vi "Post_Process_Profile_Remote.vi"(1 "Results Plotter Rows":string[][](array[string]), 2 "Raw Data files to PP":path[](array[path]), 3 "Current Results filenames":path[](array[path])) -> ()   [LabVIEW 2010]
uses:
  Globals/Constants_global.vi
panel:
  in  "User Specific":refnum<vi>
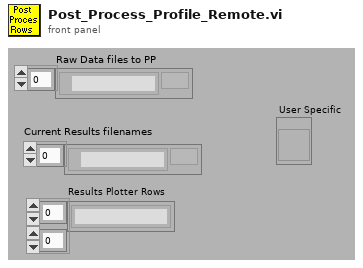
[diagram p1: front panel]
types:
  T1 = enum32{"Bad", "Idle", "Run top level", "Running"}
  T2 = enum16{"A single file", "Original Results Filenames with _PP", "Current Results Filenames"}
  T3 = enum16{"Left Button", "Center Button", "Right Button", "Window Close"}
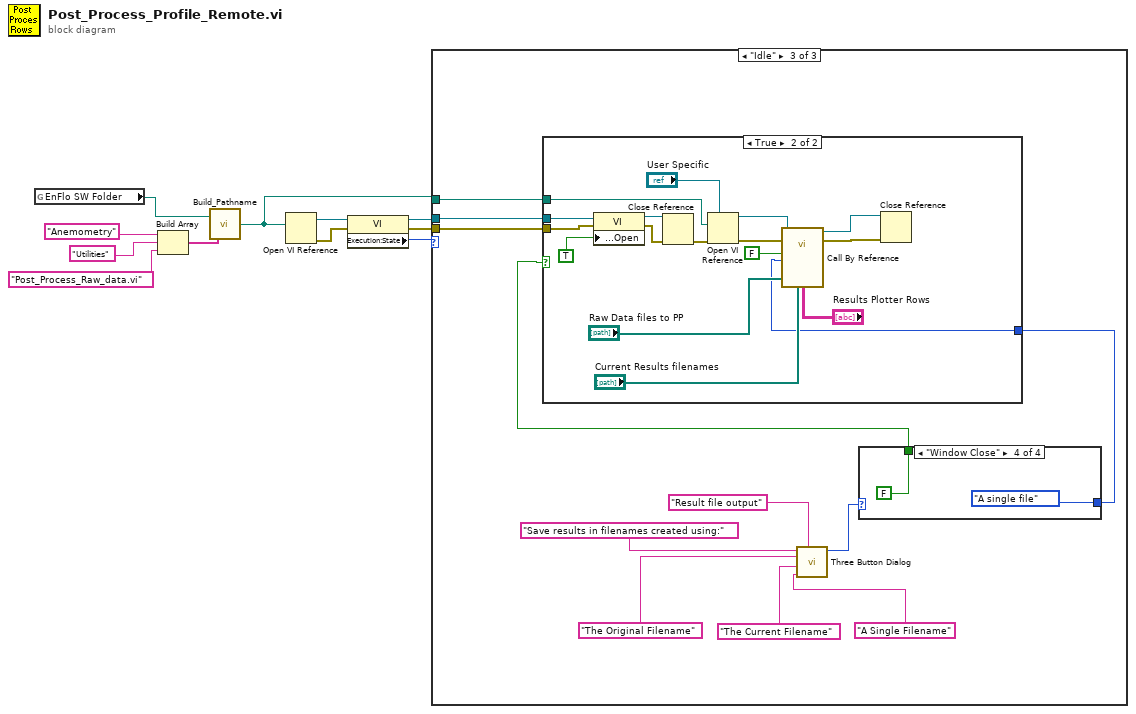
[diagram p0: block diagram]
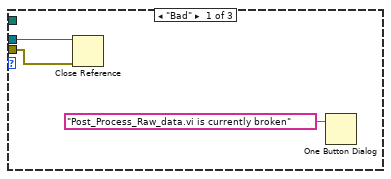
[diagram p2: hidden frame]
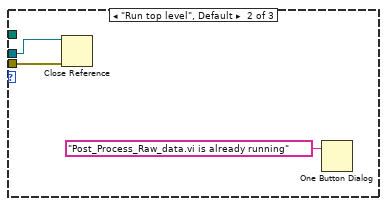
[diagram p3: hidden frame]
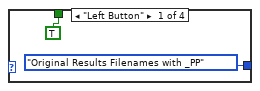
[diagram p5: hidden frame]
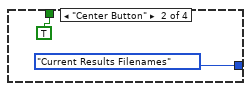
[diagram p6: hidden frame]
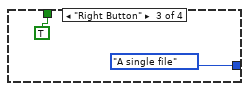
[diagram p7: hidden frame]
diagram:
  n1 = global read "Constants_global.vi" "EnFlo SW Folder"() -> (w11:path)
  n2 = Build Array("Anemometry", "Utilities", "Post_Process_Raw_data.vi") -> (w10:string[])
  n3 = call "Build_Pathname.vi"("Output Array"=w10, "Pathname"=w11) -> ("Appended path"=w2:path)
  n4 = Open VI Reference(vi path=w2) -> (vi reference=w6:refnum<vi>, error out=w7:errorcluster)  [unwired: 1 in, 4 out]
  n5 = property class="VI"(reference=w6, error in=w7) -> (reference out=w4:refnum<vi>, error out=w3:errorcluster, "Execution:State"=w5:T1)
  n6 = case shown="\"Idle\"" w5 {
    tunnel: w4 -> [w13 w16 w28]
    tunnel: w3 -> [w12 w15 w27]
    tunnel: w2 -> [_ _ w26]
    frame "Bad" {
      n7 = Close Reference(reference=w13, error in (no error)=w12) -> ()  [unwired: 1 out]
      n8 = One Button Dialog(message="Post_Process_Raw_data.vi is currently broken") -> ()  [unwired: 2 out]
    }
    frame "Run top level", Default {
      n9 = Close Reference(reference=w16, error in (no error)=w15) -> ()  [unwired: 1 out]
      n10 = One Button Dialog(message="Post_Process_Raw_data.vi is already running") -> ()  [unwired: 2 out]
    }
    frame "Idle" {
      n11 = call <vilib>:"Three Button Dialog.vi"("Window Title (\"\")"="Result file output" ("Window Title (\"\")"), "Right Button Text (\"Cancel\")"="A Single Filename" ("Left Button Text (\"Yes\")"), "Center Button Text (\"No\")"="The Current Filename" ("Left Button Text (\"Yes\")"), "Left Button Text (\"Yes\")"="The Original Filename" ("Left Button Text (\"Yes\")"), "message"="Save results in filenames created using:") -> ("Which Button?"=w20:T3)  [unwired: 6 out]
      n12 = case shown="\"Window Close\"" w20 {
        tunnel: [T2."Original Results Filenames with _PP" ("Save results to") T2."Current Results Filenames" ("Save results to") T2."A single file" ("Save results to") T2."A single file" ("Save results to")] -> w19
        tunnel: [TRUE TRUE TRUE FALSE] -> w18
        frame "Left Button" {
        }
        frame "Center Button" {
        }
        frame "Right Button" {
        }
        frame "Window Close" {
        }
      }
      n13 = case shown="True" w18 {
        tunnel: w28 -> [_ w45]
        tunnel: w27 -> [_ w44]
        tunnel: w26 -> [_ w43]
        tunnel: w19 -> [_ w30]
        frame False {
        }
        frame True {
          n14 = property class="VI"(reference=w45, error in=w44, "Front Panel Window:Open"=TRUE) -> (reference out=w39:refnum<vi>, error out=w38:errorcluster)
          n15 = Close Reference(reference=w39, error in (no error)=w38) -> (error out=w37:errorcluster)
          n16 = Open VI Reference(type specifier VI Refnum (for type only)="User Specific", vi path=w43, error in (no error)=w37) -> (vi reference=w35:refnum<vi>, error out=w34:errorcluster)  [unwired: 3 out]
          n17 = call-by-ref "?"(reference=w35, error in=w34, "Select Plug Ins"=FALSE, "Save results to"=w30, "Selected files"="Raw Data files to PP", "Current Results filenames"="Current Results filenames", "Results Plotter Rows"="Results Plotter Rows") -> (reference out=w41:refnum<vi>, error out=w40:errorcluster)  [unwired: 11 in]
          n18 = Close Reference(reference=w41, error in (no error)=w40) -> ()  [unwired: 1 out]
        }
      }
    }
  }
